vi "Set Mixer.vi"(8 "error in (no error)":errorcluster, 10 "Mixer":dbl(knob) scale=0.0..100.0, 11 "Feeder Actor.lvlib:Mixer.lvclass":refnum<class "Mixer.lvclass">) -> (0 "error out":errorcluster, 3 "Actor out":refnum<class "Actor.lvclass">)   [LabVIEW 2018, in "Feeder Actor.lvlib" / "Mixer.lvclass"]
uses:
  Mixer.lvclass
  C:/Program Files/National Instruments/LabVIEW 2018/vi.lib/ActorFramework/Actor/Actor.lvclass
  <vilib>/ActorFramework/Actor/Actor.lvclass
  Mixer.lvclass/Mixer.ctl
  <vilib>/DAQmx/write.llb/DAQmx Write (Counter Frequency 1Chan 1Samp).vi
  <vilib>/DAQmx/miscellaneous.llb/DAQmx Fill In Error Info.vi
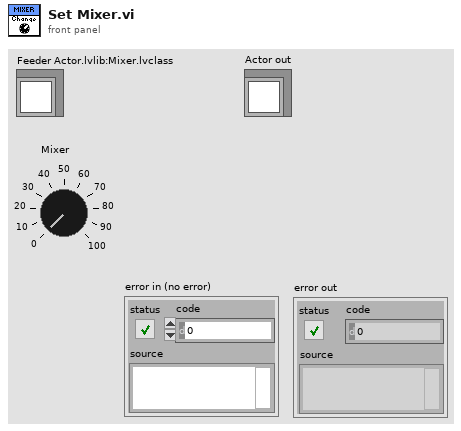
[diagram p1: front panel]
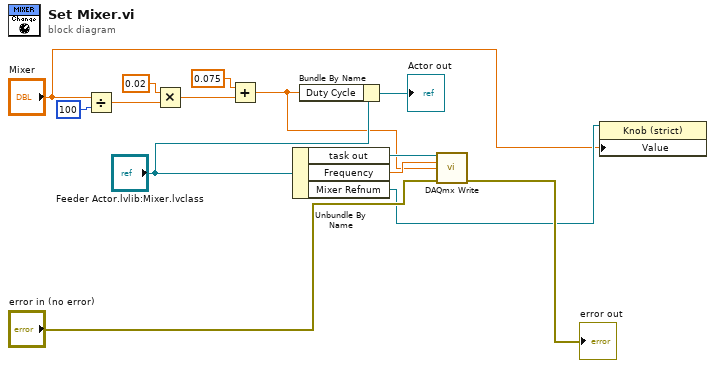
[diagram p0: block diagram]
diagram:
  n1 = Divide(x="Mixer", y=i16 100) -> (x/y=w11:dbl)
  n2 = Multiply(x=0.02, y=w11) -> (x*y=w8:dbl)
  n3 = Add(x=0.075, y=w8) -> (x+y=w6:dbl)
  n4 = Unbundle By Name("Feeder Actor.lvlib:Mixer.lvclass") -> ("task out"=w14:refnum<k21>, "Frequency"=w13:dbl, "Mixer Refnum"=w2:refnum<vi>)
  n5 = Bundle By Name(cluster="Feeder Actor.lvlib:Mixer.lvclass", "Duty Cycle"=w6) -> (→"Actor out":refnum<class "Mixer.lvclass">)
  n6 = call-poly <vilib>:"DAQmx Write.vi"("task/channels in"=w14, "frequency"=w13, "duty cycle"=w6, "error in"="error in (no error)") -> ("error out"=→"error out":errorcluster)  [unwired: 9 in, 2 out]
  n7 = property class="Knob (strict)"(reference=w2, "Value"="Mixer") -> ()  [unwired: 1 in, 2 out]
